vi "Test Test Finder Find Correct Number of Methods.vi"(8 "error in (no error)":errorcluster, 11 "Test Finder In":refnum<class "Test Finder.lvclass">) -> (0 "error out":errorcluster, 3 "Test Finder Out":refnum<class "Test Finder.lvclass">)   [LabVIEW 2020, in "LUnit Tests.lvlib" / "Test Finder.lvclass"]
uses:
  Test Finder.lvclass
  C:/Program Files (x86)/National Instruments/LabVIEW 2020/vi.lib/Asteme/LUnit/Test Case.lvclass
  Test Dummys/Descending Test Test Case/Descending Test Test Case.lvclass
  Test Finder.lvclass/Test Finder.ctl
  source/Framework/Helper Classes/Test Finder/Test Finder.lvclass/Test Finder.ctl
  <vilib>/Asteme/LUnit/Test Case.lvclass/Test Case.ctl
  <vilib>/Asteme/LUnit/LUnit Assertion Result.lvclass/LUnit Assertion Result.ctl
  <vilib>/Asteme/LUnit/LUnit Test Case Result.lvclass/LUnit Test Case Result.ctl
  <vilib>/Asteme/LUnit/LUnit Method Result.lvclass/LUnit Method Result.ctl
  <vilib>/Asteme/LUnit/Palette/Pass.vi
  <vilib>/Asteme/LUnit/Palette/Fail.vi
  <vilib>/Asteme/LUnit/Variant to string.vi
  <vilib>/Asteme/LUnit/Set Assertion Type.vi
  <vilib>/Asteme/LUnit/Add test result.vi
  <vilib>/Asteme/LUnit/LUnit Write Passed.vi
  <vilib>/Asteme/LUnit/LUnit Write Message.vi
  <vilib>/Asteme/LUnit/LUnit Write Description.vi
  <vilib>/Asteme/LUnit/LUnit Write Assertion Type.vi
  <vilib>/Asteme/LUnit/LUnit Record Assertion Result.vi
  <vilib>/Asteme/LUnit/LUnit Aggregate Assertion Results.vi
  <vilib>/Asteme/LUnit/Assertion Result/LUnit Read Status.vi
  <vilib>/Asteme/LUnit/LUnit Read Message.vi
  <vilib>/Asteme/LUnit/LUnit Read Description.vi
  <vilib>/Asteme/LUnit/Method Result/LUnit Merge Status.vi
  <vilib>/Asteme/LUnit/LUnit Concatenate result strings.vi
  source/Framework/Helper Classes/Test Finder/Public/Accessors/Read Test Method Names.vi
  <vilib>/Utility/Data Type/Get Type Information.vi
  <vilib>/Utility/LVClass/Get LV Class Name.vi
  source/Framework/Helper Classes/Test Finder/Test Finder.lvclass
  <vilib>/Asteme/LUnit/LUnit Assertion Result.lvclass
  <vilib>/Asteme/LUnit/Test Case.lvclass
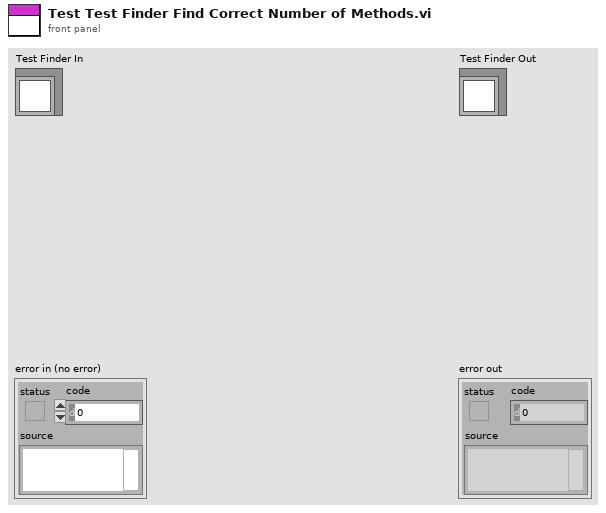
[diagram p1: front panel]
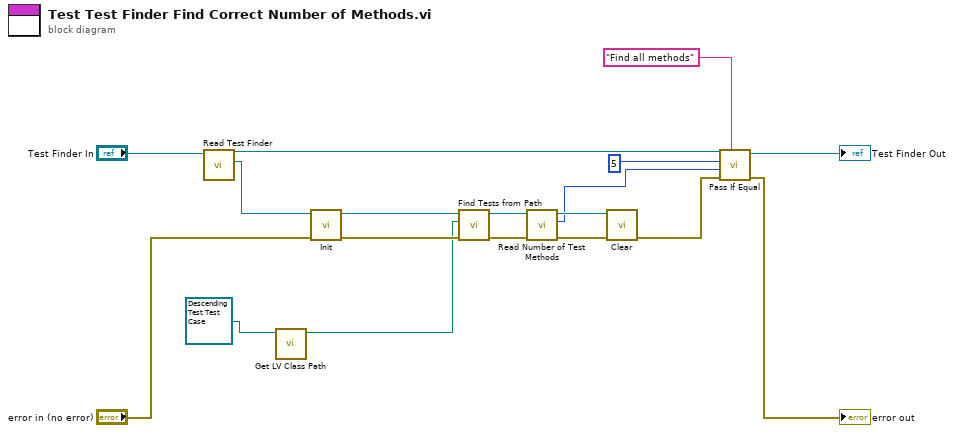
[diagram p0: block diagram]
diagram:
  n1 = call "Read Test Finder.vi"("Test Finder In"="Test Finder In") -> ("Test Finder.lvclass"=w17:refnum<class "Test Finder.lvclass">, "Test Finder Out"=w7:refnum<class "Test Finder.lvclass">)  [unwired: 8 in, 1 out]
  n2 = call <vilib>:"Get LV Class Path.vi"("object"=refnum<class "Descending Test Test Case.lvclass"> refnum ("Descending Test Test Case.lvclass")) -> ("class path"=w13:path)  [unwired: 9 in, 1 out]
  n3 = call-dynamic "Init.vi"("error in (no error)"="error in (no error)", "Test Finder in"=w17) -> ("error out"=w15:errorcluster, "Test Finder out"=w16:refnum<class "Test Finder.lvclass">)  [unwired: 8 in]
  n4 = call-dynamic "Find Tests from Path.vi"("error in (no error)"=w15, "Project or Class Path"=w13, "Test Case Finder In"=w16) -> ("error out"=w10:errorcluster, "Test Case Finder Out"=w12:refnum<class "Test Finder.lvclass">)  [unwired: 7 in]
  n5 = call "Read Number of Test Methods.vi"("error in (no error)"=w10, "Test Finder In"=w12) -> ("error out"=w9:errorcluster, "Number of Test Methods found"=w1:i32, "Test Finder Out"=w11:refnum<class "Test Finder.lvclass">)  [unwired: 7 in]
  n6 = call "Clear.vi"("error in (no error)"=w9, "Test Finder in"=w11) -> ("error out"=w5:errorcluster)  [unwired: 8 in, 1 out]
  n7 = call <vilib>:"Pass If Equal.vi"("Description"="Find all methods", "error in (no error)"=w5, "Actual"=w1, "Expected"=5 ("x"), "LUnit Test Case In"=w7) -> ("error out"=→"error out":errorcluster, "LUnit Test Case Out"=→"Test Finder Out":refnum<class "Test Finder.lvclass">)  [unwired: 5 in]
